vi "Signal Gen test.vi"() -> ()   [LabVIEW 2020]
doc: "This example demonstrates how to use the Signal Generator function, which you can use to generate sine, sawtooth, square, and random waveforms."
uses:
  <vilib>/Simulation/Scripting/Companion Diagram/SimConfigNode/SimParams.ctl
  <vilib>/Simulation/Scripting/Companion Diagram/SimConfigNode/_simSolvers.ctl
  <vilib>/Simulation/Implementation/Shared/SIMSCR Execution Mode.ctl
  <vilib>/Platform/TimedLoop/XDataNode/timing_clust.ctl
  <vilib>/Platform/TimedLoop/XDataNode/nitl_modes.ctl
  <vilib>/Platform/TimedLoop/XDataNode/wakeup.ctl
  <vilib>/Simulation/Param Hierarchy/Typedefs/SIMPH Param Control Actions.ctl
  <vilib>/Simulation/Implementation/Shared/NILVSim_ParamChanged.vi
  <vilib>/Simulation/Implementation/Shared/NILVSim_FinishedLate.vi
  <vilib>/Simulation/Implementation/Shared/NILVSIM_BeginStep.vi
  <vilib>/Simulation/DataSources/Implementation/NILVSim Signal Generator.llb/SIM Signal Generator (scalar).vi
  <vilib>/Simulation/SignalDisplay/Implementation/NILVSim Time Waveform.llb/SIM Time Waveform (scalar).vi
  <vilib>/Simulation/Utility/Implementation/SIM Halt.vi
  <vilib>/Simulation/Implementation/Shared/NILVSim_Manager.vi
  <vilib>/Utility/error.llb/Clear Errors.vi
  <vilib>/Simulation/Implementation/Shared/NILVSim_FinalizeModel.vi
  <vilib>/Simulation/Implementation/Shared/SIM Unbundle Sim Info.vi
  <vilib>/Simulation/Implementation/Shared/SIMSH Read Queue.vi
  <vilib>/Simulation/Implementation/Shared/NILVSim_Initialize.vi
  <vilib>/Simulation/Utility/Implementation/NILVSim Get Time and IsAcceptedStep.vi
  <vilib>/Simulation/Implementation/Shared/NILVSim_GetModelError.vi
  <vilib>/Simulation/Implementation/Shared/SIM Bundle Sim Info.vi
  <vilib>/Simulation/Scripting/Companion Diagram/SimConfigNode/SimDog.xnode
  <vilib>/Platform/TimedLoop/XDataNode/XDataNode.xnode
  <vilib>/Simulation/Implementation/XNodeFramework/SimXNode/SimX.xnode
  <vilib>/Platform/TimedLoop/XDataNode/XDNodeRunTimeDep.lvlib
  <vilib>/Simulation/Implementation/Shared/NI_SIM_Implementation.lvlib
panel:
  in  "stop 2":bool
  in  "signal type 2":enum16{"Sine", "Square", "Sawtooth", "Random"}(ring)
  in  "amplitude 2":dbl=1.0
  in  "frequency 2":dbl=0.5
  in  "phase 2":dbl
  out "Waveform Chart 2":waveform(dbl)(graph)
  out "Waveform Chart":waveform(dbl)(graph)
  in  "phase":dbl
  in  "frequency":dbl=0.5
  in  "amplitude":dbl=1.0
  in  "signal type":enum16{"Sine", "Square", "Sawtooth", "Random"}(ring)
  in  "stop":bool
  # "Overview: This example demonstrates how to use the Signal Generator function, which you can use to generate sine, sawtooth, square, and random waveforms.\nInstructions:\n1. Setup the initial and final value and run the VI.\n2. Change values of controls and analyze the response on the chart."
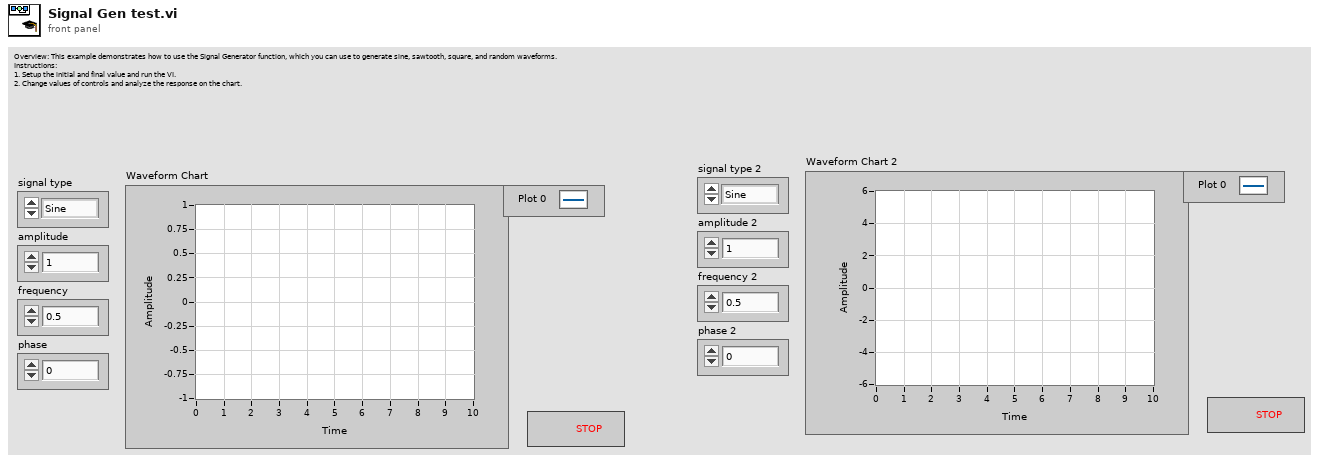
[diagram p1: front panel]
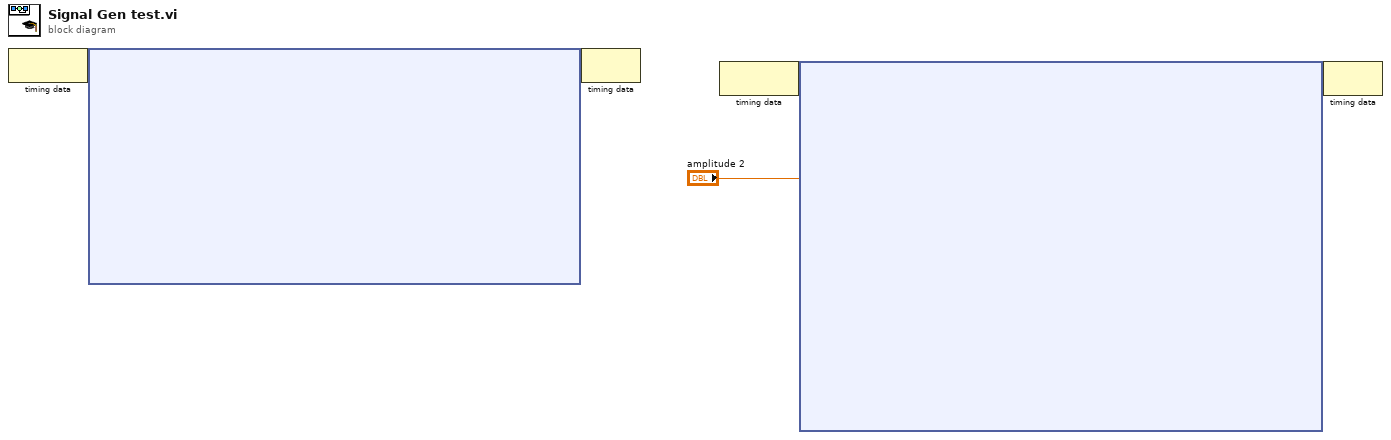
[diagram p0: block diagram]
diagram:
  n1 = node-c288() -> (w5:variant)  [unwired: 1 in]
  n2 = node-c254 ("Control & Simulation Loop")(w5) -> (w4:variant)
  n3 = node-c288(w4) -> ()  [unwired: 1 out]
  n4 = node-c288() -> (w3:variant)  [unwired: 1 in]
  n5 = node-c254 ("Control & Simulation Loop 2")(w3, "amplitude 2") -> (w2:variant)
  n6 = node-c288(w2) -> ()  [unwired: 1 out]
